vi "PRL SIGNAL Create Waveform.vi"(7 "Index":i32, 10 "Analog Signals":sgl[][](array[numeric]), 11 "Timestamp":timestamp[](array[timestamp])) -> (3 "output waveform":waveform(sgl))   [LabVIEW 2013, in "PMU Recorder Light.lvlib"]
uses:
  PMU Recorder Light.lvlib
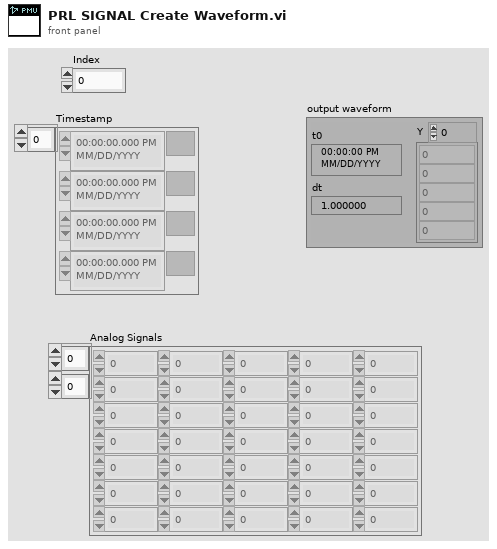
[diagram p1: front panel]
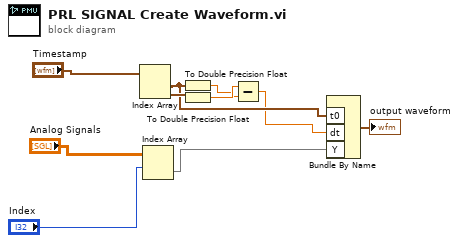
[diagram p0: block diagram]
diagram:
  n1 = Index Array(array="Timestamp") -> (element #1=w6:timestamp, element #2=w9:timestamp)  [unwired: 2 in]
  n2 = Index Array(array="Analog Signals", index (row)="Index") -> (element=w2:sgl[])  [unwired: 1 in]
  n3 = To Double Precision Float(number=w6) -> (double precision float=w7:dbl)
  n4 = To Double Precision Float(number=w9) -> (double precision float=w8:dbl)
  n5 = Subtract(x=w8, y=w7) -> (x-y=w5:dbl)
  n6 = Bundle By Name("t0"=w6, "dt"=w5, "Y"=w2) -> (→"output waveform":waveform(sgl))  [unwired: 1 in]
